vi "RPI2 Main.vi"() -> ()   [LabVIEW 2014]
uses:
  User Defined/I2C_Platform_Selector.ctl
  <vilib>/Platform/TimedLoop/XDataNode/timing_clust.ctl
  <vilib>/Platform/TimedLoop/XDataNode/nitl_modes.ctl
  <vilib>/Platform/TimedLoop/XDataNode/wakeup.ctl
  <vilib>/MakerHub/LINX/Public/Peripherals/Digital/Digital Write 1 Chan.vi
  <vilib>/MakerHub/LINX/Public/Peripherals/Digital/Digital Write N Chans.vi
  <vilib>/MakerHub/LINX/Private/Local IO/LinxDigitalWrite.vi
  <vilib>/MakerHub/LINX/Public/Utilities/Check Channel.vi
  <vilib>/MakerHub/LINX/Private/Local IO/Handle Errors.vi
  <vilib>/MakerHub/LINX/Public/Utilities/Open Local.vi
  <vilib>/MakerHub/LINX/Private/Utilties/Generate Error.vi
  <vilib>/platform/TimedLoop/XDataNode/XDataNode.xnode
  <vilib>/MakerHub/LINX/LMH-LINX.lvlib
  <vilib>/MakerHub/LINX/Private/Type Defs/Peripherals/SPI/SPI Bit Order.ctl
  <vilib>/MakerHub/LINX/Private/Type Defs/Peripherals/SPI/SPI Mode.ctl
  <vilib>/MakerHub/LINX/Private/Type Defs/Peripherals/SPI/SPI Configuration.ctl
  <vilib>/MakerHub/LINX/Private/Type Defs/Peripherals/SPI/SPI CS Logic Level.ctl
  <vilib>/MakerHub/LINX/Public/Peripherals/SPI/SPI CS Config.ctl
  <vilib>/MakerHub/LINX/Public/Peripherals/Digital/Digital Read 1 Chan.vi
  <vilib>/Platform/TimedLoop/XDataNode/XDNodeRunTimeDep.lvlib
panel:
  out "error out 2":errorcluster
  out "length":i32
  out "error out":errorcluster
  out "mV out":dbl
  out "Array":i32[](array[numeric]) format="%.0x"
  out "max value":dbl format="%#_f"
  in  "Stop Button 3":bool
  out "Error Out":errorcluster
  out "Waveform Chart":dbl[](graph)
  in  "DI Channel":u8
  in  "DO Channel":u8=24
  in  "Stop Button":bool
  out "Converted Voltage (V)":dbl
  out "10-bit ADC Code":u16 format="%.0x"
  in  "stop":bool
  out "Temperature (degC)":dbl
  # "Raspberry Pi 2 Blink!\n\nUse this VI to blink and LED connected to the specified digital output channel.\n1. Connect an LED to pin 7 and ground as shown in the image below.\n2. Click the round LED control below to blink the LED.\n\nFor more details on the Raspberry Pi 2 LINX channels visit labviewmakerhub.com/linx/raspberry-pi-2\nVisit labviewmakerhub.com/forums/linx to get help and share your projects."
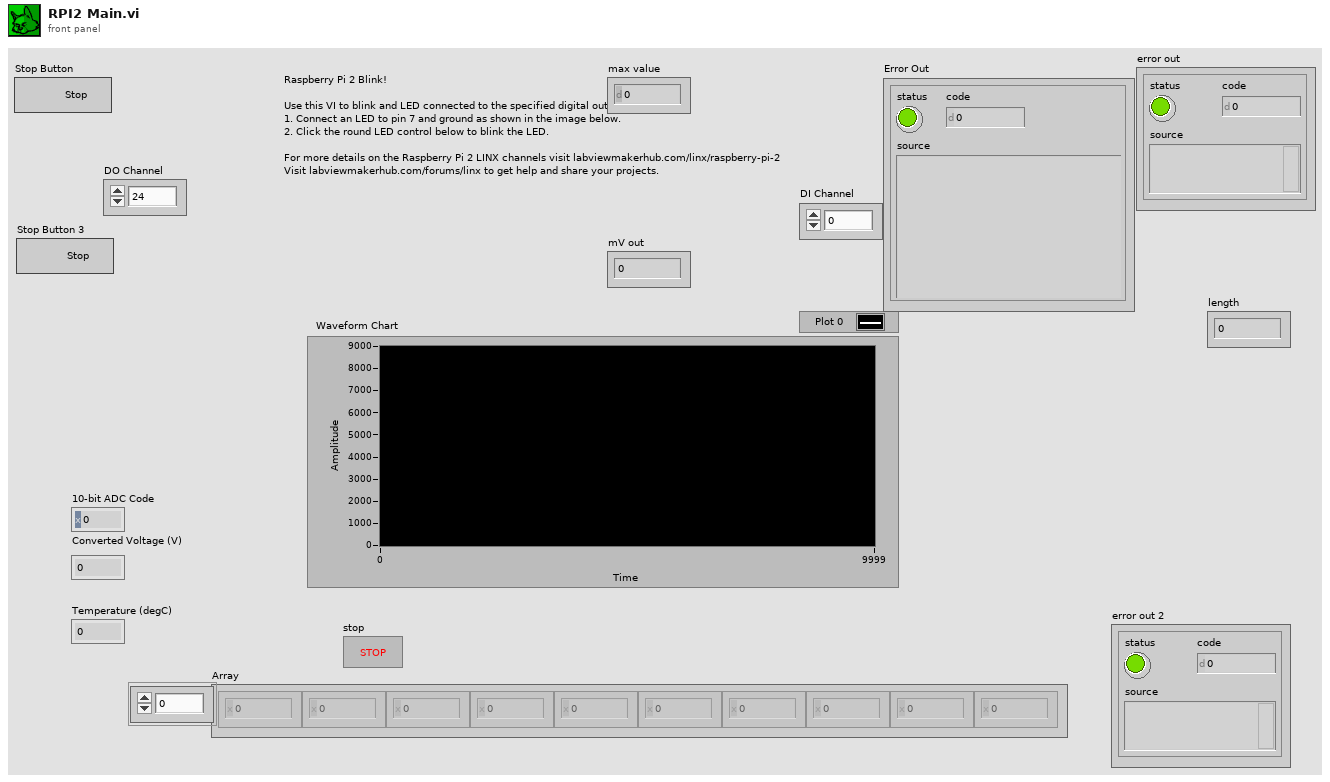
[diagram p1: front panel]
types:
  T1 = typedef "I2C_Platform_Selector.ctl" = enum16{"ESP8266-I2C", "Raspberry Pi-I2C"}
  T2 = cluster{"ADS1015-Channel Selector":enum8{"DIFF-AI0-AI1", "DIFF-AI0-AI3", "DIFF-AI1-AI3", "DIFF-AI2-AI3", "Single Ended - AI0", "Single Ended - AI1", "Single Ended - AI2", "Single Ended - AI3"}, "ADS1015 -Gain & Scale":enum8{"FS=+/-6.144 V", "FS=+/-4.096 V", "FS=+/-2.048 V", "FS=+/-1.024 V", "FS=+/-0.512 V", "FS=+/-0.256-A V", "FS=+/-0.256-B V", "FS=+/-0.256-C V"}, "ADS1015- Acquire Mode":enum16{"Continuous Conversion Mode", "Single Shot Mode"}, "ADS1015 Sample Rate":enum8{"128 SPS", "250 SPS", "490 SPS", "920 SPS", "1600 SPS", "2400 SPS", "3300 SPS", "3300 SPS A"}}
  T3 = typedef "LMH-LINX.lvlib/SPI CS Config.ctl" = cluster{"CS Channel":u8, "CS Logic Level":T4}
  T4 = typedef "LMH-LINX.lvlib/SPI CS Logic Level.ctl" = enum8{"Active Low", "Active High"}
  T5 = typedef "LMH-LINX.lvlib/SPI Configuration.ctl" = cluster{"Clock Frequency":u32, "Bit Order":T6, "SPI Mode":T7}
  T6 = typedef "LMH-LINX.lvlib/SPI Bit Order.ctl" = enum8{"LSb First", "MSb First"}
  T7 = typedef "LMH-LINX.lvlib/SPI Mode.ctl" = enum8{"Mode 0", "Mode 1", "Mode 2", "Mode 3"}
  T8 = enum16{"CH0 (0=IN+, 1=IN-)", "CH1 (1=IN+, 0=IN-)", "CH2 (2=IN+, 3=IN-)", "CH3 (3=IN+, 2=IN-)", "CH4 (4=IN+, 5=IN-)", "CH5 (5=IN+, 4=IN-)", "CH6 (6=IN+, 7=IN-)", "CH7 (7=IN+, 6=IN-)"}
  T9 = typedef "LMH-LINX.lvlib/LINX Ref.ctl" = cluster{"IO":T10, "Interface":T11, "LINX Device Config":T12}
  T10 = typedef "LMH-LINX.lvlib/Platform.ctl" = enum16{"Remote", "Local"}
  T11 = typedef "LMH-LINX.lvlib/Interface.ctl" = enum16{"Serial", "TCP"}
  T12 = typedef "LMH-LINX.lvlib/Device.lvlib/LINX Device Config.ctl" = cluster{"Interface":T11, "COM Port":refnum<visa-resource-name>, "TCP Configuration":T13, "Device Family":u8, "Device ID":u8, "Device Name":string, "TCP Ref":refnum<k5>, "Channels":T14}
  T13 = typedef "LMH-LINX.lvlib/Device.lvlib/TCP Config.ctl" = cluster{"IP Address":string, "Port":u16}
  T14 = typedef "LMH-LINX.lvlib/Channels.ctl" = cluster{"DI":u8[], "DO":u8[], "AI":u8[], "AO":u8[], "PWM":u8[], "QE":u8[], "UART":u8[], "I2C 2":u8[], "SPI":u8[], "CAN":u8[], "Servo":u8[], "AI Ref (V)":dbl, "AI Resolution (Bits)":u8, "AO Ref (V)":dbl, "AO Resolution (Bits)":u8}
  T15 = enum8{"FS=+/-6.144 V", "FS=+/-4.096 V", "FS=+/-2.048 V", "FS=+/-1.024 V", "FS=+/-0.512 V", "FS=+/-0.256-A V", "FS=+/-0.256-B V", "FS=+/-0.256-C V"}
  T16 = typedef "XDNodeRunTimeDep.lvlib/timing_clust.ctl" = cluster{"Expected End [f-1]":u64, "Actual End [f-1]":u64, "Finished Late? [f-1]":bool, "Expected End [i-1]":u64, "Actual End [i-1]":u64, "Finished Late? [i-1]":bool, "Expected Start [i]":u64, "Actual Start [i]":u64, "Expected Start [f]":u64, "Actual Start [f]":u64, "Source Name":string, "Structure Name":string, "Period":i64, "Deadline":i64, "Offset":i64, "Start":i64, "Priority":i32, "Timeout":i32, "Mode":T17, "Wakeup Reason":T18, "Error":errorcluster, "Source Type":string, "Secondary Source Type":string, "Global End Time":u64, "Global Start Time":u64, "Frame Duration":u64, "Iteration Duration":u64, "Assigned CPU":i32, "I/O Scan Engine Mode":u32}
  T17 = typedef "XDNodeRunTimeDep.lvlib/nitl_modes.ctl" = enum32{"No Change", "Process missed periods, maintain original phase", "Discard missed periods, maintain original phase", "Process missed periods, ignore original phase", "Discard missed periods, ignore original phase"}
  T18 = typedef "XDNodeRunTimeDep.lvlib/wakeup.ctl" = enum32{"Normal", "Aborted", "Asynchronous wakeup", "Timing source error", "Timed loop error", "Timeout"}
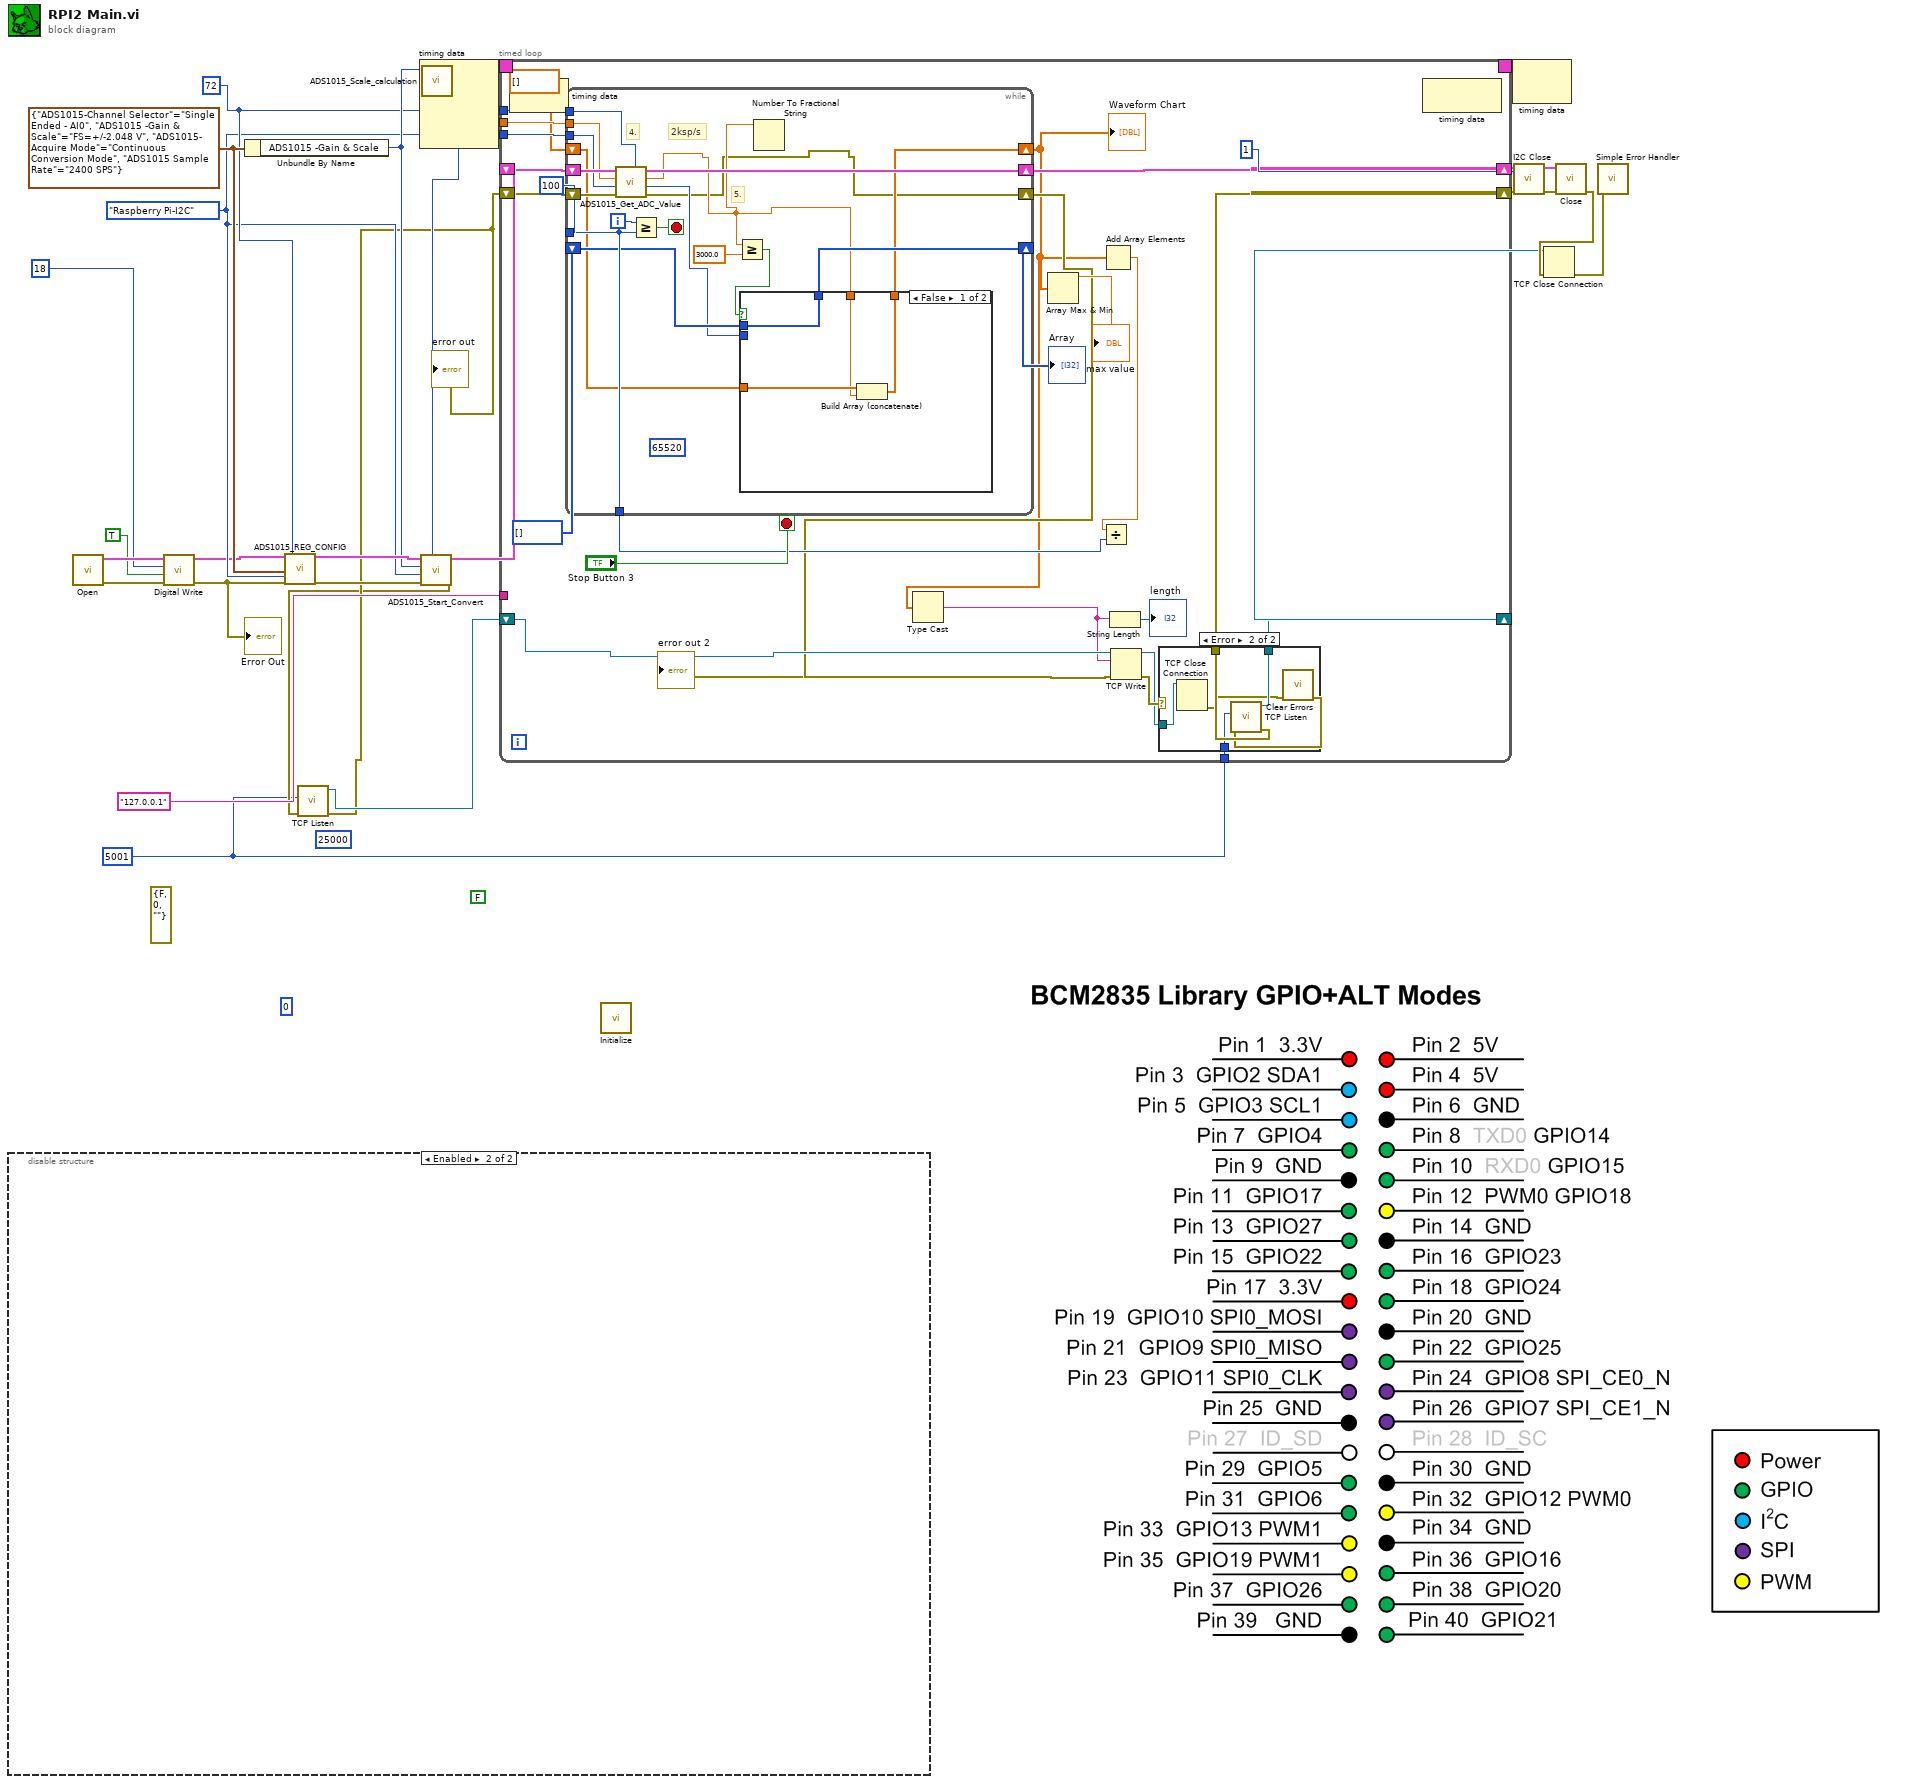
[diagram p0: block diagram]
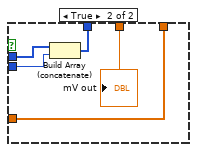
[diagram p3: hidden frame]
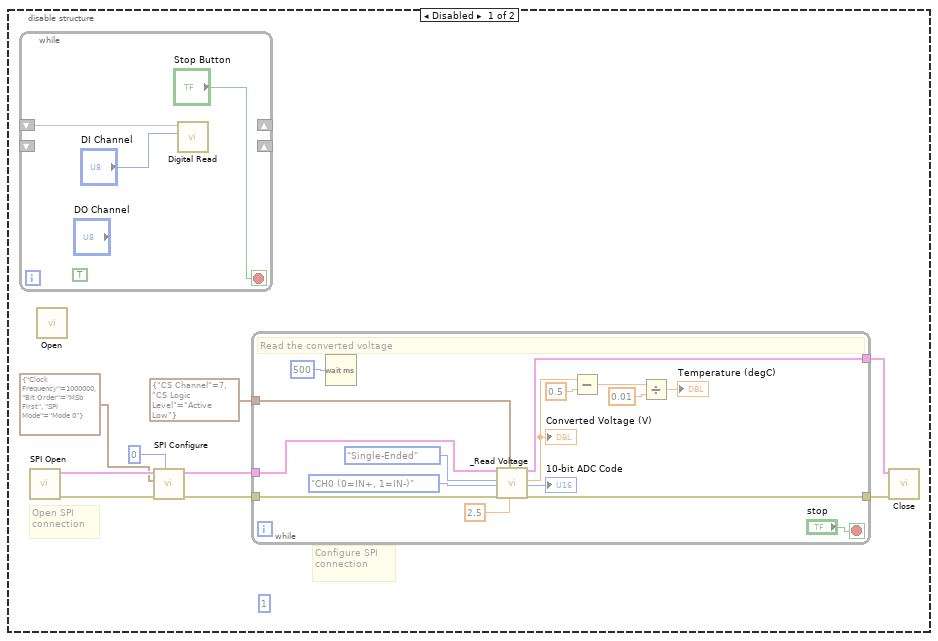
[diagram p4: hidden frame]
diagram:
  (unwired) 25000 ("timeout ms (25000)")
  (unwired) FALSE
  (unwired) errorcluster {"status"=FALSE, "code"=0, "source"=""} ("error in")
  w3 = u16 5001 ("port")
  (unwired) 0 ("bytes written")
  w17 = I2C_Platform_Selector."Raspberry Pi-I2C" ("I2C_Channel_platform")
  w18 = u8 72 ("I2C Slave Address (0)")
  w25 = T2 {"ADS1015-Channel Selector"=enum."Single Ended - AI0", "ADS1015 -Gain & Scale"=enum."FS=+/-2.048 V", "ADS1015- Acquire Mode"=enum."Continuous Conversion Mode", "ADS1015 Sample Rate"=enum."2400 SPS"} ("ADS1015 Reg Config")
  n1 = disable-structure shown="Enabled" {
    frame Disabled {
      (unwired) u8 1 ("SPI Channel (0)")
      # "Configure SPI connection"
      # "Open SPI connection"
      n2 = while {
        shift-right: [w54] -> w31
        shift-left: _ -> [w48]
        shift-right: [w50] -> w30
        shift-left: _ -> [w53]
        stop <- "Stop Button" stop-if-true
        w51 = TRUE ("Output Value")
        n3 = call-poly <vilib>:"Digital Read.vi"("DI Channel"="DI Channel", "LINX Resource"=w48) -> ("DI Value"=w45:bool, "LINX Resource"=w47:T9)  [unwired: 7 in, 1 out]
      }
      n4 = call <vilib>:"SPI Open.vi"() -> ("Error Out"=w39:errorcluster, 3:"LINX Resource"=w40:T9, "Error In"=w33:errorcluster, 11:"LINX Resource"=w35:T9)  [unwired: 8 in]
      n5 = call-poly <vilib>:"Open.vi"() -> ("Error Out"=w34:errorcluster, "LINX Resource"=w36:T9)  [unwired: 9 in, 1 out]
      n6 = call <vilib>:"SPI Configure.vi"("SPI Channel (0)"=u8 0, "Error In"=w39, "SPI Configuration"=T5 {"Clock Frequency"=1000000, "Bit Order"=enum."MSb First", "SPI Mode"=enum."Mode 0"}, "LINX Resource"=w40) -> ("Error Out"=w41:errorcluster, "LINX Resource"=w42:T9)  [unwired: 5 in, 1 out]
      n7 = while {
        tunnel: w41 -> [w70]
        tunnel: w42 -> [w67]
        tunnel: [w68] -> w43
        tunnel: [w66] -> w44
        tunnel: T3 {"CS Channel"=7, "CS Logic Level"=enum."Active Low"} ("CS Configuration") -> [w65]
        stop <- "stop" stop-if-true
        # "Read the converted voltage"
        n8 = Wait (ms)(milliseconds to wait=u32 500) -> ()  [unwired: 1 out]
        n9 = call "_Read Voltage.vi"("LINX Resource in"=w67, "Single-Diff Select (Diff)"=enum16{"Differential", "Single-Ended"}."Single-Ended", "Channel Select (CH0)"=T8."CH0 (0=IN+, 1=IN-)", "error in (no error)"=w70, "CS Configuration"=w65, "Vref (3.3V)"=2.5) -> ("LINX Resource out"=w66:T9, "Converted Voltage (V)"=w55:dbl, "12-bit ADC Code"=→"10-bit ADC Code":u16, "error out"=w68:errorcluster)  [unwired: 8 in, 2 out]
        "Converted Voltage (V)" <- w55
        n10 = Subtract(x=w55, y=0.5) -> (x-y=w58:dbl)
        n11 = Divide(x=w58, y=0.01) -> (x/y=→"Temperature (degC)":dbl)
      }
      n12 = call <vilib>:"Close.vi"("Error In"=w43, "LINX Resource"=w44) -> ()  [unwired: 9 in, 1 out]
    }
    frame Enabled {
    }
  }
  n13 = call-poly <vilib>:"Open.vi"() -> ("Error Out"=w12:errorcluster, "LINX Resource"=w16:T9)  [unwired: 9 in, 1 out]
  n14 = call-poly <vilib>:"Digital Write.vi"("Error In"=w12, "Output Value"=TRUE, "DO Channel"=u8 18 ("DI Channel 2"), "LINX Resource"=w16) -> ("Error Out"=w7:errorcluster, "LINX Resource"=w15:T9)  [unwired: 6 in]
  "Error Out" <- w7
  n15 = Unbundle By Name(w25) -> ("ADS1015 -Gain & Scale"=w24:T15)
  n16 = call "ADS1015_REG_CONFIG.vi"("LINX Resource in"=w15, "ADS1015 Reg Config"=w25, "I2C_Channel_platform"=w17, "Error In"=w7, "I2C Slave Address (0)"=w18) -> ("LINX Resource out"=w28:T9, "Error Out"=w29:errorcluster)  [unwired: 13 in]
  n17 = node-c288() -> (w2:T16)  [unwired: 4 in]
  n18 = call "ADS1015_Start_Convert.vi"("I2C Slave Address (0)"=w18, "error in (no error)"=w29, "I2C_Channel_platform"=w17, "Scale mV"=w24, "LINX Resource in"=w28) -> ("error out"=w4:errorcluster, "LINX Resource out"=w27:T9)  [unwired: 4 in, 1 out]
  n19 = call <vilib>:"TCP Listen.vi"("error in (no error)"=w4, "port"=w3) -> ("error out"=w5:errorcluster, "connection ID"=w6:refnum<k5>)  [unwired: 5 in, 3 out]
  "error out" <- w5
  n20 = call "ADS1015_Scale_calculation.vi"("ADS1015 -Gain & Scale"=w24) -> ("Scale Value (mV)"=w26:dbl)  [unwired: 10 in]
  n21 = timed-loop {
    tunnel: w26 -> [w93]
    tunnel: w18 -> [w90]
    tunnel: w17 -> [w89]
    shift-right: [w73] -> w20
    shift-left: w5 -> [w81]
    shift-right: [w92] -> w22
    shift-left: w27 -> [w94]
    tunnel: "127.0.0.1" ("address") -> [_]
    shift-right: [w74] -> w9
    shift-left: w6 -> [w80]
    tunnel: w3 -> [w72]
    timing: w2 -> [_]
    timing-out: [_] -> w1
    stop <- "Stop Button 3" stop-if-true
    n22 = node-c288() -> ()  [unwired: 1 in, 1 out]
    n23 = while {
      shift-right: [w119] -> w92
      shift-left: w94 -> [w120]
      shift-right: [w105] -> w79
      shift-left: w81 -> [w122]
      shift-right: [w110] -> w71
      shift-left: dbl[] [] -> [w111]
      tunnel: w90 -> [w118]
      tunnel: w93 -> [w117]
      tunnel: 100 ("y") -> [w114]
      tunnel: w89 -> [w116]
      tunnel: [w114] -> w86
      shift-right: [w112] -> w82
      shift-left: i32[] [] -> [w113]
      i -> [w121]
      stop <- w115 stop-if-true
      (unwired) 65520 ("Numeric Control")
      # "2ksp/s"
      # "5."
      # "4."
      n24 = call "ADS1015_Get_ADC_Value.vi"("I2C Slave Address (0)"=w118, "error in (no error)"=w122, "I2C_Channel_platform"=w116, "Scale Value (mV)"=w117, "LINX Resource in"=w120) -> ("error out"=w105:errorcluster, "(hi.lo)"=w109:u16, "mV out"=w106:dbl, "LINX Resource"=w119:T9)  [unwired: 3 in]
      n25 = Greater Or Equal?(x=w121, y=w114) -> (x >= y?=w115:bool)
      n26 = Greater Or Equal?(x=w106, y=3000.0) -> (x >= y?=w107:bool)
      n27 = case shown="False" w107 {
        tunnel: w113 -> [w126 w131]
        tunnel: [w126 w130] -> w112
        tunnel: w109 -> [_ w129]
        tunnel: w111 -> [w125 w128]
        tunnel: w106 -> [w124 w127]
        tunnel: [w123 w128] -> w110
        frame False {
          n28 = Build Array (concatenate)(w125, w124) -> (w123:dbl[])
        }
        frame True {
          n29 = Build Array (concatenate)(w131, w129) -> (w130:i32[])
          "mV out" <- w127
        }
      }
      n30 = Number To Fractional String(number=w106) -> ()  [unwired: 3 in, 1 out]
    }
    "Waveform Chart" <- w71
    "Array" <- w82
    n31 = Type Cast(x=w71) -> (*(type *) &x=w77:string)  [unwired: 1 out]
    n32 = Array Max & Min(array=w71) -> (max value=→"max value":dbl)  [unwired: 3 out]
    n33 = Add Array Elements(numeric array=w71) -> (sum=w85:dbl)
    n34 = Divide(x=w85, y=w86) -> ()  [unwired: 1 out]
    n35 = String Length(string=w77) -> (length=→"length":i32)
    n36 = TCP Write(connection ID=w80, data in=w77, error in (no error)=w79) -> (connection ID out=w75:refnum<k5>, error out=w76:errorcluster)  [unwired: 2 out]
    "error out 2" <- w76
    n37 = case shown="Error" w76 {
      selector: w76 -> [w97 _]
      tunnel: w75 -> [w98 w101]
      tunnel: [w98 w104] -> w74
      tunnel: [w97 w103] -> w73
      tunnel: w72 -> [_ w102]
      frame No Error {
      }
      frame Error {
        n38 = TCP Close Connection(connection ID=w101) -> (error out=w100:errorcluster)  [unwired: 2 in, 1 out]
        n39 = call <vilib>:"Clear Errors.vi"("error in (no error)"=w100) -> ("error out"=w99:errorcluster)  [unwired: 5 in, 1 out]
        n40 = call <vilib>:"TCP Listen.vi"("error in (no error)"=w99, "port"=w102) -> ("error out"=w103:errorcluster, "connection ID"=w104:refnum<k5>)  [unwired: 5 in, 3 out]
      }
    }
    n41 = node-c288() -> ()  [unwired: 1 in, 1 out]
  }
  n42 = call <vilib>:"Initialize.vi"() -> ()  [unwired: 10 in, 2 out]
  n43 = node-c288(w1) -> ()  [unwired: 1 out]
  n44 = call <vilib>:"I2C Close.vi"("I2C Channel (0)"=u8 1, "Error In"=w20, "LINX Resource"=w22) -> ("Error Out"=w19:errorcluster, "LINX Resource"=w21:T9)  [unwired: 7 in]
  n45 = call <vilib>:"Close.vi"("Error In"=w19, "LINX Resource"=w21) -> ("Error Out"=w11:errorcluster)  [unwired: 9 in]
  n46 = TCP Close Connection(connection ID=w9, error in (no error)=w11) -> (error out=w10:errorcluster)  [unwired: 1 in, 1 out]
  n47 = call <vilib>:"Simple Error Handler.vi"("error in (no error)"=w10) -> ()  [unwired: 4 in, 5 out]
